vi "start listen.vi"(8 "error in":errorcluster, 11 "server acceptor in":refnum<class "server acceptor.lvclass">) -> (0 "error out":errorcluster)   [LabVIEW 2016, in "server acceptor.lvclass"]
uses:
  server acceptor.lvclass
  C:/Users/IEUser/Desktop/libasynclvtls/tls classes/connection creator/connection creator.lvclass
  connection creator.lvclass/connection creator.ctl
  server acceptor.lvclass/server acceptor.ctl
  connection creator.lvclass
  dllwrapper/async tls dl.lvlib
panel:
  out "error out 2":errorcluster
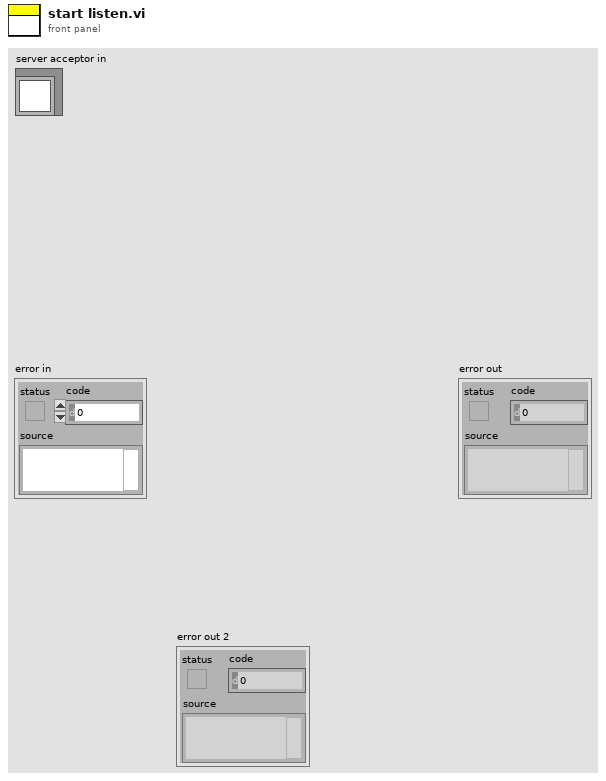
[diagram p1: front panel]
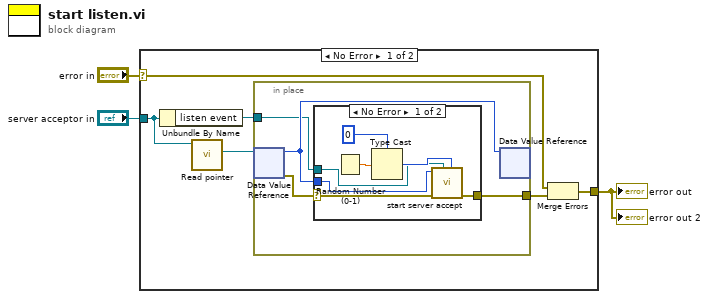
[diagram p0: block diagram]
diagram:
  n1 = case shown="No Error" "error in" {
    selector: "error in" -> [w8 w22]
    tunnel: [w7 w22] -> w1
    tunnel: "server acceptor in" -> [w5 _]
    frame No Error {
      n2 = Unbundle By Name(w5) -> ("listen event"=w4:refnum<user-event>)
      n3 = call "Read pointer.vi"("connection creator in"=w5) -> ("pointer"=w9:refnum<data-value>)  [unwired: 10 in]
      n4 = in-place {
        in-place-border: [w12] -> w6
        in-place-border: w4 -> [w10]
        n5 = in-place-dvr #1(w9) -> (w11:u64, w13:errorcluster)
        n6 = case shown="No Error" w13 {
          selector: w13 -> [w20 w21]
          tunnel: [w19 w21] -> w12
          tunnel: w11 -> [w18 _]
          tunnel: w10 -> [w14 _]
          frame No Error {
            n7 = Random Number (0-1)() -> (number: 0 to 1=w17:dbl)
            n8 = Type Cast(type=u32 0 ("request id"), x=w17) -> (*(type *) &x=w15:u32)
            n9 = call "start server accept.vi"("id"=w15, "event"=w14, "error in"=w20, "acceptor"=w18) -> ("error out"=w19:errorcluster)  [unwired: 7 in]
          }
          frame Error {
          }
        }
        n10 = in-place-dvr #1(w11) -> ()  [unwired: 2 out]
      }
      n11 = Merge Errors(w8, w6) -> (w7:errorcluster)
    }
    frame Error {
    }
  }
  "error out" <- w1
  "error out 2" <- w1
